vi "Replace 2D Array.vi"(8 "Elements to Replace":dbl[][](array[numeric]), 9 "Replacement Column":i32, 10 "Replacement Row":i32, 11 "Current Array":dbl[][](array[numeric])) -> (3 "output array":dbl[][](array[numeric]))   [LabVIEW 2012]
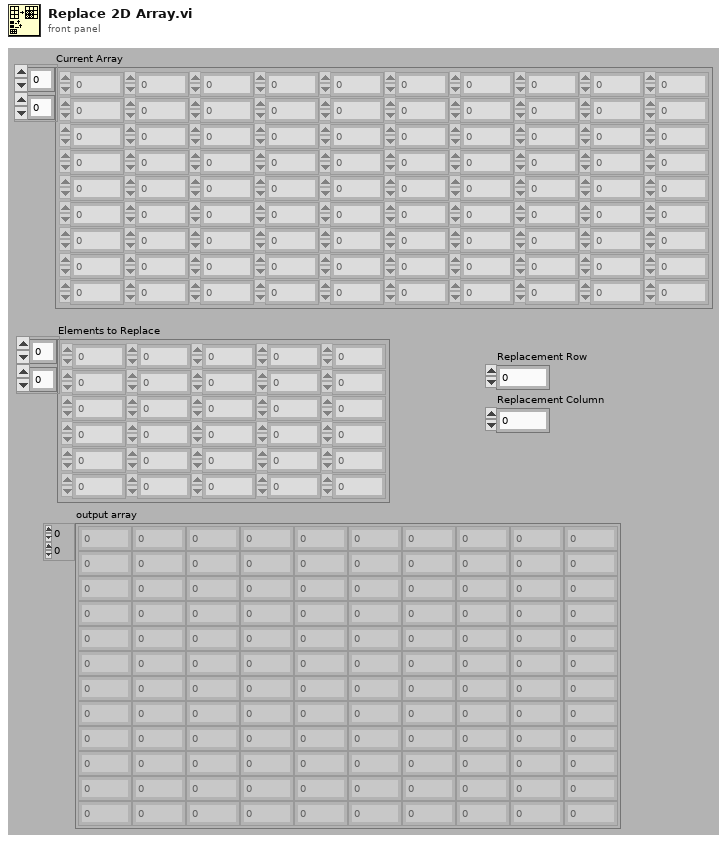
[diagram p1: front panel]
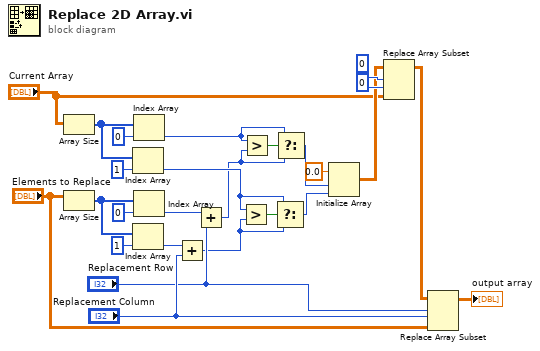
[diagram p0: block diagram]
diagram:
  n1 = Array Size(array="Current Array") -> (size(s)=w21:i32[])
  n2 = Array Size(array="Elements to Replace") -> (size(s)=w25:i32[])
  n3 = Index Array(array=w21, index=1) -> (element=w18:i32)
  n4 = Index Array(array=w25, index=1) -> (element=w10:i32)
  n5 = Index Array(array=w21, index=0) -> (element=w16:i32)
  n6 = Index Array(array=w25, index=0) -> (element=w7:i32)
  n7 = Add(x=w10, y="Replacement Column") -> (x+y=w5:i32)
  n8 = Add(x=w7, y="Replacement Row") -> (x+y=w6:i32)
  n9 = Greater?(x=w18, y=w5) -> (0:w19:bool)
  n10 = Greater?(x=w16, y=w6) -> (0:w17:bool)
  n11 = Select(t=w18, s=w19, f=w5) -> (s? t:f=w3:i32)
  n12 = Select(t=w16, s=w17, f=w6) -> (s? t:f=w4:i32)
  n13 = Initialize Array(0.0, w4, w3) -> (w14:dbl[][])
  n14 = Replace Array Subset(array=w14, new element="Current Array", index (row)=0, index (col)=0 ("disabled index (col)")) -> (w13:dbl[][])
  n15 = Replace Array Subset(array=w13, new element="Elements to Replace", index (row)="Replacement Row", index (col)="Replacement Column") -> (→"output array":dbl[][])
